vi "ma_Process RMS for N Blocks.vi"(6 "reset":bool, 7 "window for RMS":T2(ring)=enum."Hanning", 8 "time signal data (samples)":dbl[][](array[numeric]) format="%0.2p", 10 "averaging type":enum16{"Linear", "Exponential"}(ring), 11 "state info":T1 {"buffer" format="%0.2f"; "timestamp" format="%<%.4X>T"; "dt history" format="%0.2f"; "t0 history" format="%<%I:%M:%S%4u %p>T"; "exp TC (samples)" format="%0.2f"; "RMS history" format="%0.2f"; "DC history" format="%0.2f"}) -> (2 "RMS value data":dbl[](array[numeric]) format="%0.2f", 3 "state info":T1 {"buffer" format="%0.2f"; "timestamp" format="%<%.4X>T"; "dt history" format="%0.2f"; "t0 history" format="%<%I:%M:%S%4u %p>T"; "exp TC (samples)" format="%0.2f"; "RMS history" format="%0.2f"; "DC history" format="%0.2f"})   [LabVIEW 2020, in "NI_MAPro.lvlib"]
uses:
  NI_MAPro.lvlib
  NI_AALPro.lvlib
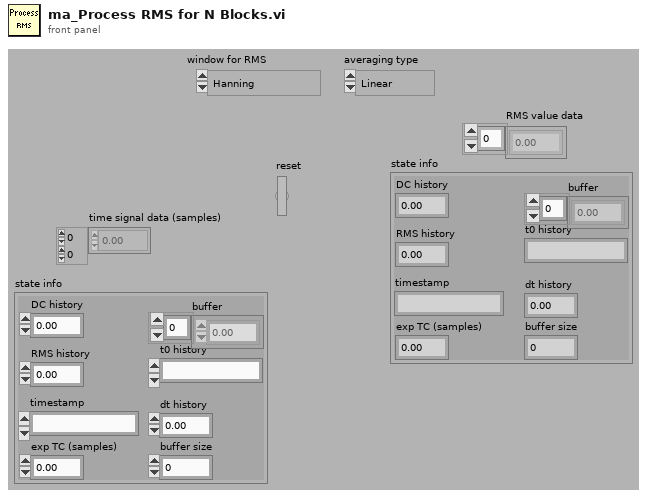
[diagram p1: front panel]
types:
  T1 = cluster{"DC history":dbl, "RMS history":dbl, "exp TC (samples)":dbl, "buffer size":i32, "t0 history":timestamp, "dt history":dbl, "timestamp":timestamp, "buffer":dbl[]}
  T2 = enum16{"Rectangular (none)", "Hanning", "Low side lobe"}
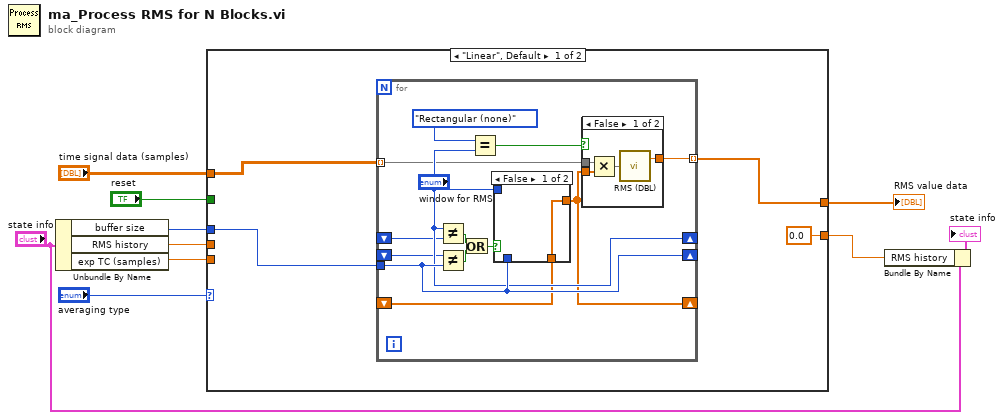
[diagram p0: block diagram]
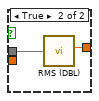
[diagram p2: hidden frame]
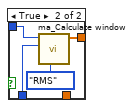
[diagram p3: hidden frame]
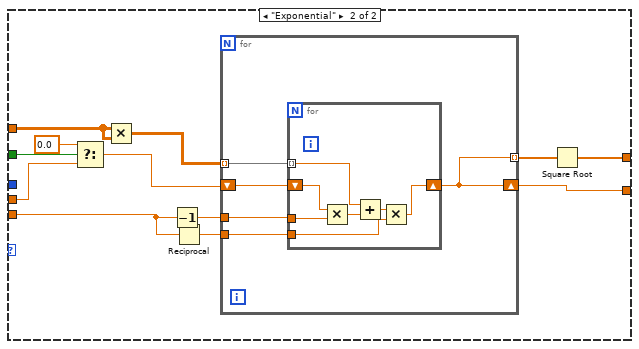
[diagram p4: hidden frame]
diagram:
  n1 = Unbundle By Name("state info") -> ("buffer size"=w6:i32, "RMS history"=w4:dbl, "exp TC (samples)"=w5:dbl)
  n2 = case shown="\"Linear\", Default" "averaging type" {
    tunnel: w6 -> [w14 _]
    tunnel: [w11 w39] -> w8
    tunnel: w5 -> [_ w47]
    tunnel: "time signal data (samples)" -> [w12 w41]
    tunnel: [0.0 w44] -> w2
    tunnel: "reset" -> [_ w43]
    tunnel: w4 -> [_ w40]
    frame "Linear", Default {
      n3 = for {
        tunnel: [w25] -> w11 mode=indexing
        tunnel: w14 -> [w27]
        tunnel: w12 -> [w24] mode=indexing
        shift-right: ["window for RMS"] -> _
        shift-left: _ -> [w16]
        shift-right: [w27] -> _
        shift-left: _ -> [w17]
        shift-right: [w18] -> _
        shift-left: _ -> [w15]
        n4 = Not Equal?(x="window for RMS", y=w16) -> (x != y?=w23:bool)
        n5 = Not Equal?(x=w17, y=w27) -> (x != y?=w22:bool)
        n6 = Or(x=w23, y=w22) -> (x .or. y?=w21:bool)
        n7 = Equal?(x=T2."Rectangular (none)", y="window for RMS") -> (x = y?=w19:bool)
        n8 = case shown="False" w21 {
          tunnel: "window for RMS" -> [_ w38]
          tunnel: w27 -> [_ w37]
          tunnel: [w34 w35] -> w18
          tunnel: w15 -> [w34 _]
          frame False {
          }
          frame True {
            n9 = call "ma_Calculate window.vi"("scaled for"=enum16{"DC", "RMS"}."RMS", "array size"=w37, "window"=w38) -> ("Window data"=w35:dbl[])  [unwired: 8 in]
          }
        }
        n10 = case shown="False" w19 {
          tunnel: w24 -> [w31 w33]
          tunnel: [w30 w32] -> w25
          tunnel: w18 -> [w29 _]
          frame False {
            n11 = Multiply(x=w31, y=w29) -> (x*y=w28:dbl[])
            n12 = call "RMS (DBL).vi"("X"=w28) -> ("rms value"=w30:dbl)  [unwired: 1 out]
          }
          frame True {
            n13 = call "RMS (DBL).vi"("X"=w33) -> ("rms value"=w32:dbl)  [unwired: 1 out]
          }
        }
      }
    }
    frame "Exponential" {
      n14 = Select(t=0.0, s=w43, f=w40) -> (s? t:f=w48:dbl)
      n15 = Multiply(x=w41, y=w41) -> (x*y=w42:dbl[][])
      n16 = Decrement(x=w47) -> (x-1=w46:dbl)
      n17 = Reciprocal(x=w47) -> (1/x=w45:dbl)
      n18 = for {
        tunnel: w42 -> [w52] mode=indexing
        tunnel: [w51] -> w50 mode=indexing
        tunnel: w46 -> [w53]
        shift-right: [w51] -> w44
        shift-left: w48 -> [w55]
        tunnel: w45 -> [w54]
        n19 = for {
          tunnel: w52 -> [w57] mode=indexing
          shift-right: [w56] -> w51
          shift-left: w55 -> [w61]
          tunnel: w53 -> [w62]
          tunnel: w54 -> [w58]
          n20 = Multiply(x=w61, y=w62) -> (x*y=w60:dbl)
          n21 = Add(x=w57, y=w60) -> (x+y=w59:dbl)
          n22 = Multiply(x=w59, y=w58) -> (x*y=w56:dbl)
        }
      }
      n23 = Square Root(x=w50) -> (sqrt(x)=w39:dbl[])
    }
  }
  "RMS value data" <- w8
  n24 = Bundle By Name(cluster="state info", "RMS history"=w2) -> (→"state info":T1)
